vi "Setup Timing.vi"(8 "error in (no error)":errorcluster, 9 "color":T2, 10 "led":refnum<vi>, 11 "State":T1) -> (0 "error out":errorcluster, 3 "State out":T1 caption="State")   [LabVIEW 2010, in "Twinkle Button.xctl"]
doc: "本VI是为《我和LabVIEW》一书编写的示例。\n关于本书的介绍请参考网页：\nhttp://ruanqizhen.spaces.live.com/blog/cns!5852D4F797C53FB6!4310.entry"
uses:
  Twinkle Button.xctl
  Data.ctl
  State.ctl
  C:/Program Files/National Instruments/LabVIEW 2010/resource/importtools/Common/Event/NISAST Event.lvclass
  Message Data.ctl
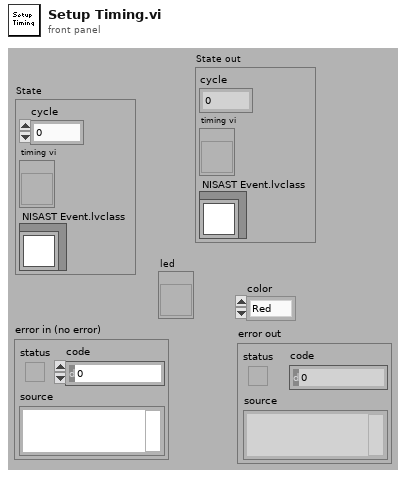
[diagram p1: front panel]
types:
  T1 = typedef "Twinkle Button.xctl/State.ctl" = cluster{"cycle":dbl, "timing vi":refnum<vi>, "NISAST Event.lvclass":refnum<class "NISAST Event.lvclass">}
  T2 = typedef "Twinkle Button.xctl/Data.ctl" = enum16{"Red", "Green", "Blue"}
  T3 = typedef "Twinkle Button.xctl/Message Data.ctl" = cluster{"cycle":dbl, "led":refnum<vi>, "color":T2}
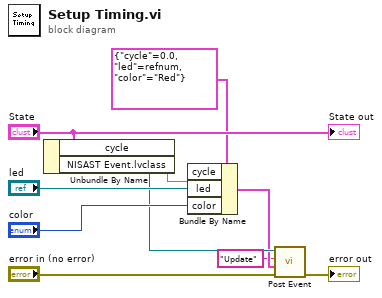
[diagram p0: block diagram]
diagram:
  n1 = Unbundle By Name("State") -> ("cycle"=w6:dbl, "NISAST Event.lvclass"=w5:refnum<class "NISAST Event.lvclass">)
  n2 = Bundle By Name(cluster=T3 {"cycle"=0.0, "led"=refnum, "color"=enum."Red"} ("data"), "cycle"=w6, "led"="led", "color"="color") -> (w3:T3)
  n3 = call-dynamic "Post Event.vi"("error in (no error)"="error in (no error)", "Event Data"=w3, "Event Name"="Update", "Event in"=w5) -> ("error out"=→"error out":errorcluster)  [unwired: 7 out]
  "State out" <- "State"
